vi "QCA - DUT Read TCP.vi"(0 "CART TCP Connection In":refnum<k5>, 11 "error in (no error)":errorcluster) -> (4 "CART TCP Connection Out":refnum<k5>, 6 "Messages Logged":string[](array[string]), 14 "Command Sent":string, 15 "error out":errorcluster)   [LabVIEW 2011]
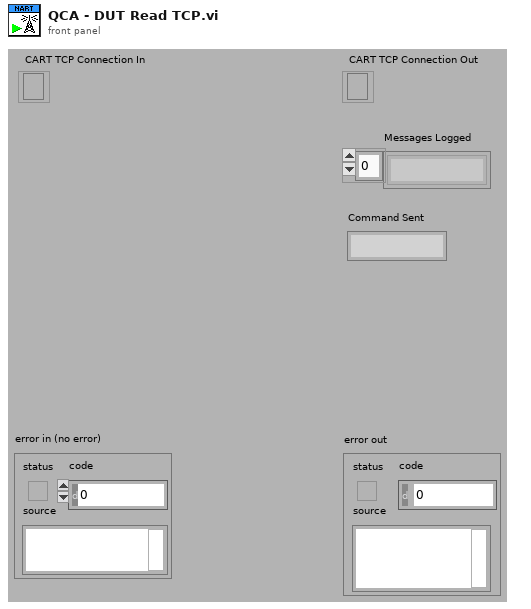
[diagram p1: front panel]
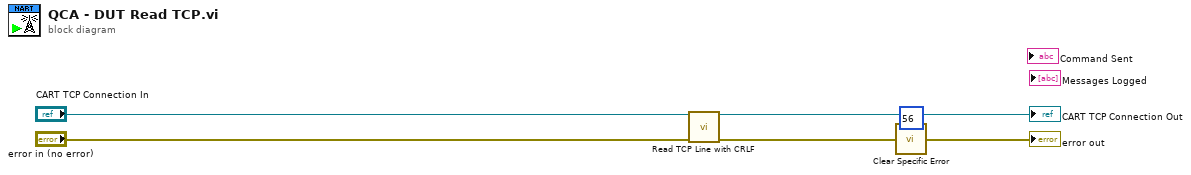
[diagram p0: block diagram]
diagram:
  n1 = call "Read TCP Line with CRLF.vi"("TCP Connection In"="CART TCP Connection In", "error in"="error in (no error)") -> ("TCP Connection Out"=→"CART TCP Connection Out":refnum<k5>, "error out"=w6:errorcluster)  [unwired: 11 in, 1 out]
  n2 = call "Clear Specific Error.vi"("Specific Error Number (0: none)"=56, "error in"=w6) -> ("error out"=→"error out":errorcluster)  [unwired: 12 in, 1 out]
